vi "FTW-JSON-Object-GetElement-Object.vi"(0 "JSON Object":refnum<class "FTW-JSON.lvclass">, 5 "Key":string, 11 "error in":errorcluster) -> (4 "JSON Root Object":refnum<class "FTW-JSON.lvclass">, 6 "JSON Sub-Object":refnum<class "FTW-JSON.lvclass">, 15 "error out":errorcluster)   [LabVIEW 2014, in "FTW-JSON.lvclass"]
uses:
  FTW-JSON.lvclass
  FTW-JSON.lvclass/FTW-JSON.ctl
  error/FTW-ERR-ThrowGenericError.vi
  error/FTW-ERR-ThrowError.vi
  error/FTW-ERR-NoErrorConstant.vi
  error/FTW-ERR-CallChain.vi
  string/FTW-STR-ReplaceWhitespace.vi
panel:
  # "Inputs"
  # "Outputs"
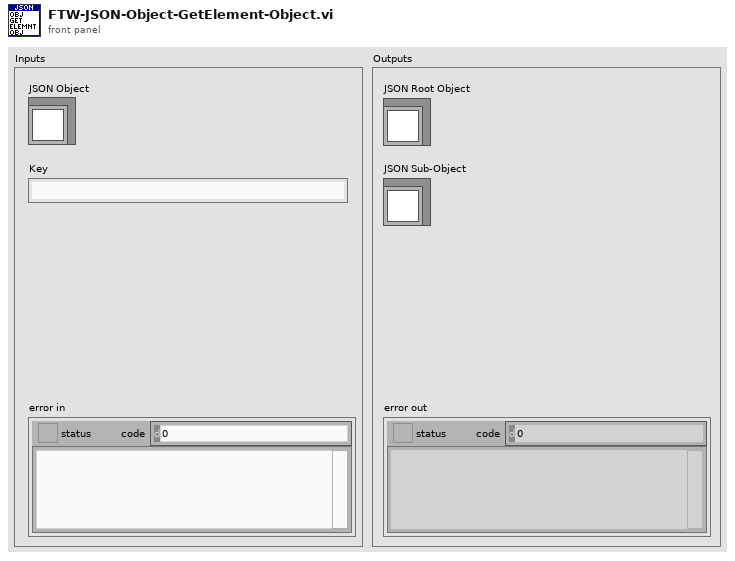
[diagram p1: front panel]
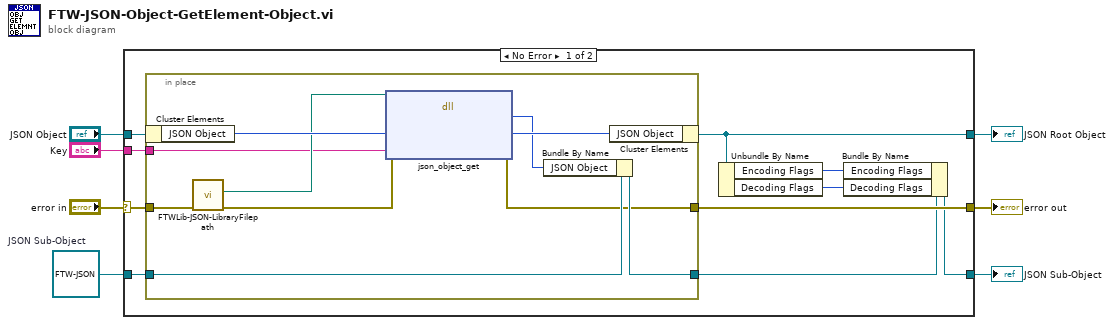
[diagram p0: block diagram]
diagram:
  w1 = refnum<class "FTW-JSON.lvclass"> refnum  # JSON Sub-Object
  n1 = case shown="No Error" "error in" {
    selector: "error in" -> [w17 w30]
    tunnel: [w16 w30] -> w7
    tunnel: [w11 w29] -> w5
    tunnel: "JSON Object" -> [w15 w29]
    tunnel: "Key" -> [w14 _]
    tunnel: [w10 w28] -> w2
    tunnel: w1 -> [w12 w28]
    frame No Error {
      n2 = in-place {
        in-place-border: w17 -> [w27]
        in-place-border: [w19] -> w16
        in-place-border: w14 -> [w21]
        in-place-border: [w25] -> w13
        in-place-border: w12 -> [w26]
        n3 = in-place-cluster #1(w15) -> ("JSON Object"=w24:i64)
        n4 = call "FTWLib-JSON-LibraryFilepath.vi"("error in"=w27) -> ("error out"=w20:errorcluster, "JSON Library Filepath"=w22:path)  [unwired: 9 in]
        n5 = dll-call lib="?" fn="json_object_get"(path in=w22, error in=w20, "JSON Object Pointer"=w24, "Element Key"=w21) -> (error out=w19:errorcluster, "JSON Element Pointer"=w18:i64, "JSON Object Pointer"=w23:i64)  [unwired: 2 in, 1 out]
        n6 = Bundle By Name(cluster=w26, "JSON Object"=w18) -> (w25:refnum<class "FTW-JSON.lvclass">)
        n7 = in-place-cluster #1("JSON Object"=w23) -> (w11:refnum<class "FTW-JSON.lvclass">)
      }
      n8 = Unbundle By Name(w11) -> ("Encoding Flags"=w9:i64, "Decoding Flags"=w8:i64)
      n9 = Bundle By Name(cluster=w13, "Encoding Flags"=w9, "Decoding Flags"=w8) -> (w10:refnum<class "FTW-JSON.lvclass">)
    }
    frame Error {
    }
  }
  "error out" <- w7
  "JSON Root Object" <- w5
  "JSON Sub-Object" <- w2
